vi "mainOCRV2.vi"() -> ()   [LabVIEW 2025]
uses:
  ocr/TextDecRecResult2L.ctl
  ocr/ocr.lvclass
  tcv/tcv.lvclass
panel:
  out "loadImgSucc":string
  out "succ 2":i32
  in  "device":enum16{"CPU", "GPU0"}(ring)
  out "InitRecDec Success":string
  out "SetDevice":string
  in  "PathImage":path=path "D:/Test/dllTest/images_2"
  out "Image":T1(plugin-control)
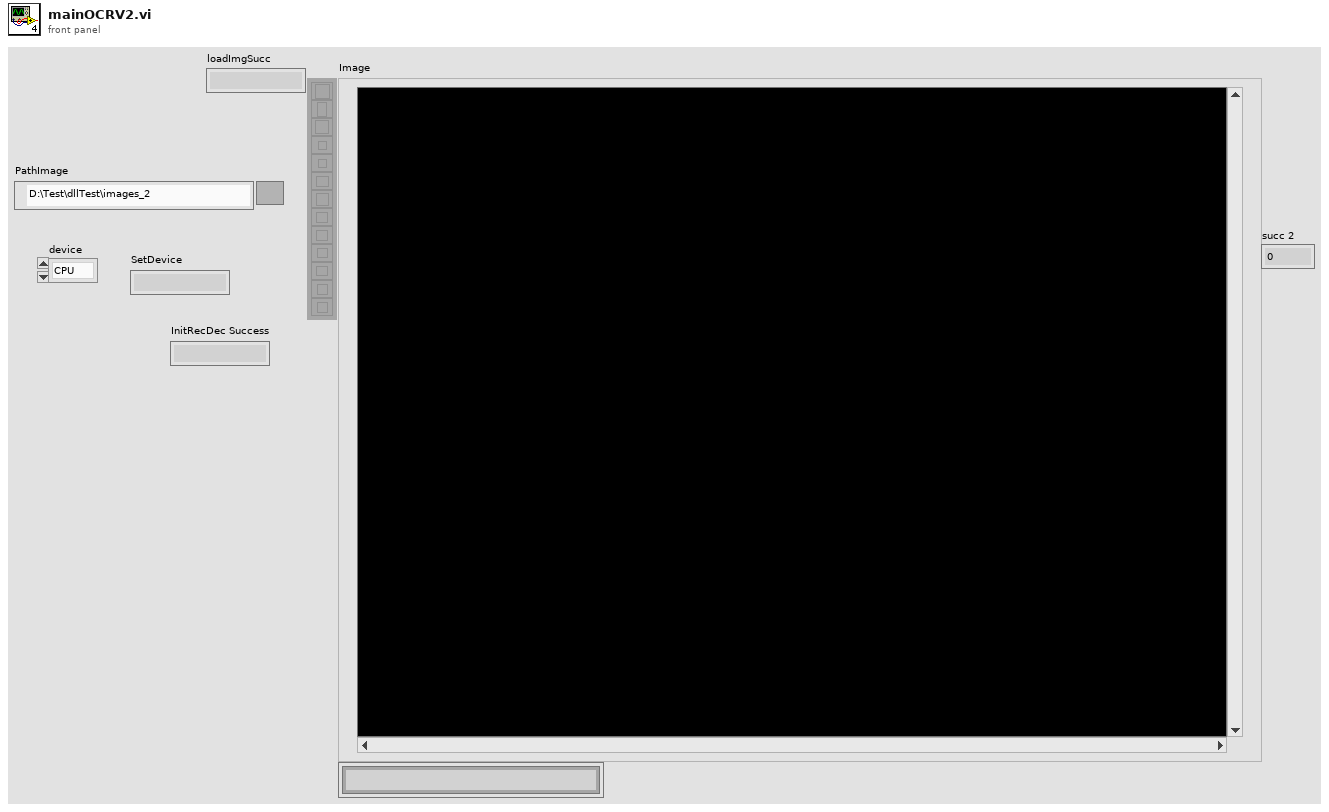
[diagram p1: front panel]
types:
  T1 = typedef "IMAQ Image.ctl" = refnum<image>
  T2 = typedef "adsOCR.lvlib/ocr.lvclass/TextDecRecResult2L.ctl" = cluster{"imgIdx":i32, "TLx":i32, "TLy":i32, "BRx":i32, "BRy":i32, "angle":sgl, "txtLen":i32}
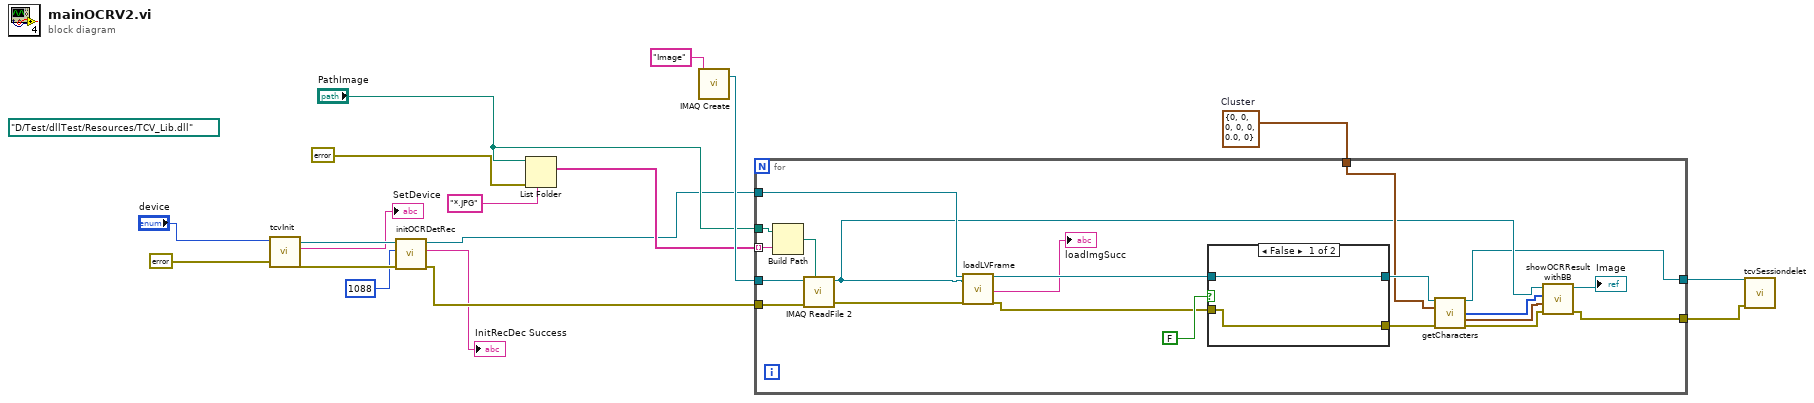
[diagram p0: block diagram]
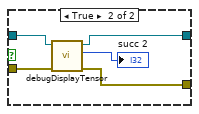
[diagram p2: hidden frame]
diagram:
  w12 = T2 {"imgIdx"=0, "TLx"=0, "TLy"=0, "BRx"=0, "BRy"=0, "angle"=0.0, "txtLen"=0}  # Cluster
  (unwired) path "D:/Test/dllTest/Resources/TCV_Lib.dll" ("path in")
  n1 = call "tcvInit.vi"("error in"=errorcluster {"status"=FALSE, "code"=0, "source"=""} ("error in (no error)"), "devices"="device") -> ("error out"=w8:errorcluster, "SetDevice"=→"SetDevice":string, "tcv out"=w9:refnum<class "tcv.lvclass">)  [unwired: 7 in]
  n2 = call "initOCRDetRec.vi"("error in (no error)"=w8, "targetSize"=1088, "tcv in"=w9) -> ("error out"=w5:errorcluster, "InitRecDec Success"=→"InitRecDec Success":string, "ocr out"=w6:refnum<class "ocr.lvclass">)  [unwired: 5 in, 1 out]
  n3 = List Folder(path="PathImage", pattern="*.JPG", error in=errorcluster {"status"=FALSE, "code"=0, "source"=""}) -> (filenames=w13:string[])  [unwired: 1 in, 3 out]
  n4 = call "IMAQ Create"("Image Name"="Image") -> ("New Image"=w18:T1)  [unwired: 4 in, 1 out]
  n5 = for {
    tunnel: "PathImage" -> [w39]
    tunnel: w18 -> [w37]
    tunnel: w12 -> [w27]
    tunnel: w13 -> [w36] mode=indexing
    tunnel: [w23] -> w4
    tunnel: w6 -> [w34]
    tunnel: w5 -> [w32]
    tunnel: [w19] -> w3
    n6 = Build Path(base path=w39, name or relative path=w36) -> (appended path=w38:path)
    n7 = call "IMAQ ReadFile 2"("File Path"=w38, "error in (no error)"=w32, "Image"=w37) -> ("error out"=w33:errorcluster, "Image Out"=w25:T1)  [unwired: 4 in, 3 out]
    n8 = call-dynamic "loadLVFrame.vi"("tcv in"=w34, "Image"=w25, "error in (no error)"=w33) -> ("tcv out"=w31:refnum<class "ocr.lvclass">, "loadImgSucc"=→"loadImgSucc":string, "error out"=w30:errorcluster)  [unwired: 13 in, 1 out]
    n9 = case shown="False" FALSE {
      tunnel: w31 -> [w41 w46]
      tunnel: w30 -> [w40 w45]
      tunnel: [w41 w44] -> w28
      tunnel: [w40 w43] -> w26
      frame False {
      }
      frame True {
        n10 = call-dynamic "debugDisplayTensor.vi"("error in (no error)"=w45, "tcv in"=w46) -> ("error out"=w43:errorcluster, "succ"=→"succ 2":i32, "tcv out"=w44:refnum<class "ocr.lvclass">)  [unwired: 6 in, 1 out]
      }
    }
    n11 = call-dynamic "getCharacters.vi"("ocr in"=w28, "Cluster"=w27, "error in (no error)"=w26) -> ("ocr out"=w19:refnum<class "ocr.lvclass">, "chars"=w21:u8[], "TextDecRecResult2L"=w20:T2[], "error out"=w22:errorcluster)  [unwired: 8 in, 1 out]
    n12 = call "showOCRResultwithBB.vi"("error in"=w22, "Array"=w20, "chars"=w21, "Image in"=w25) -> ("error out"=w23:errorcluster, "Image out"=→"Image":T1)  [unwired: 4 in]
  }
  n13 = call-dynamic "tcvSessiondelet.vi"("error in (no error)"=w4, "tcv in"=w3) -> ()  [unwired: 8 in, 2 out]
